vi "Unbundle Last Ack.vi"(11 "Last Ack":T1) -> (1 "State":string, 2 "Error":string, 3 "Ident":string)   [LabVIEW 2025]
uses:
  cmd-data event messages/source/Last Ack.ctl
  cmd-data event messages/source/Cmd-Data Event Messages.lvlib
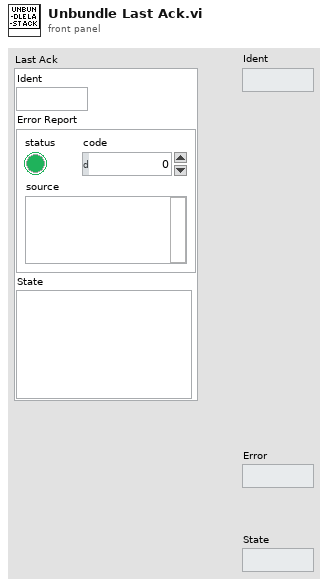
[diagram p1: front panel]
types:
  T1 = typedef "Cmd-Data Event Messages.lvlib/Last Ack.ctl" = cluster{"Ident":string, "Error Report":errorcluster, "State ":string}
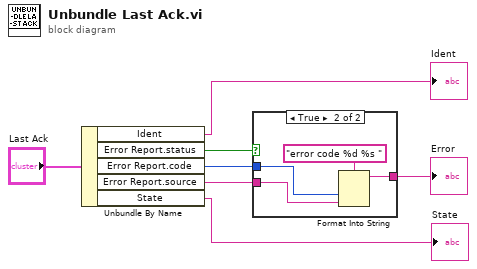
[diagram p0: block diagram]
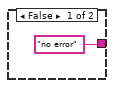
[diagram p2: hidden frame]
diagram:
  n1 = Unbundle By Name("Last Ack") -> ("Ident"=→"Ident":string, "Error Report.status"=w4:bool, "Error Report.code"=w5:i32, "Error Report.source"=w6:string, "State"=→"State":string)
  n2 = case shown="True" w4 {
    tunnel: w5 -> [_ w12]
    tunnel: w6 -> [_ w10]
    tunnel: ["no error" w9] -> w7
    frame False {
    }
    frame True {
      n3 = Format Into String(format string="error code %d %s ", w12, w10) -> (resulting string=w9:string)  [unwired: 2 in, 1 out]
    }
  }
  "Error" <- w7
